vi "stop.vi"(7 "cmd (read)":enum16{"write", "read"}(ring)=enum."read", 8 "error in (no error)":errorcluster caption="에러 입력(에러 없음)", 9 "stop":bool) -> (0 "error out":errorcluster caption="에러 출력", 1 "stop?":bool)   [LabVIEW 2020]
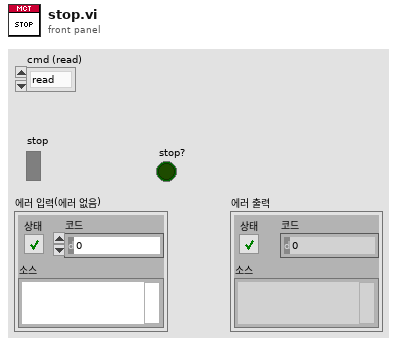
[diagram p1: front panel]
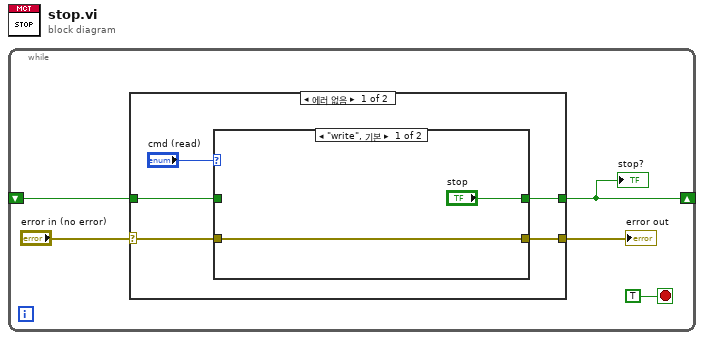
[diagram p0: block diagram]
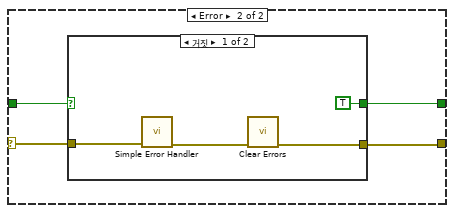
[diagram p3: hidden frame]
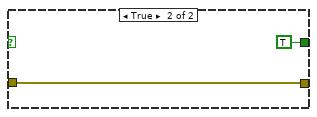
[diagram p4: hidden frame]
diagram:
  n1 = while {
    shift-right: [w1] -> _
    shift-left: _ -> [w2]
    stop <- TRUE stop-if-true
    n2 = case shown="에러 없음" "error in (no error)" {
      selector: "error in (no error)" -> [w6 w18]
      tunnel: [w9 w15] -> w1
      tunnel: w2 -> [w8 w16]
      tunnel: [w7 w17] -> w4
      frame No Error {
        n3 = case shown="\"write\", 기본" "cmd (read)" {
          tunnel: ["stop" w14] -> w9
          tunnel: w8 -> [_ w14]
          tunnel: w6 -> [w11 w13]
          tunnel: [w11 w13] -> w7
          frame "write", Default {
          }
          frame "read" {
          }
        }
      }
      frame Error {
        n4 = case shown="거짓" w16 {
          tunnel: w18 -> [w21 w24]
          tunnel: [w20 w24] -> w17
          tunnel: [TRUE TRUE] -> w15
          frame False {
            n5 = call <vilib>:"Simple Error Handler.vi"("error in (no error)"=w21) -> ("error out"=w22:errorcluster)  [unwired: 4 in, 4 out]
            n6 = call <vilib>:"Clear Errors.vi"("error in (no error)"=w22) -> ("error out"=w20:errorcluster)  [unwired: 5 in, 1 out]
          }
          frame True {
          }
        }
      }
    }
    "error out" <- w4
    "stop?" <- w1
  }
